vi "Wormgear.vi"(8 "error in (no error)":errorcluster, 11 "Buttons":bool[](array[boolean])) -> (0 "error out":errorcluster, 3 "Wormgear Power":dbl)   [LabVIEW 2016]
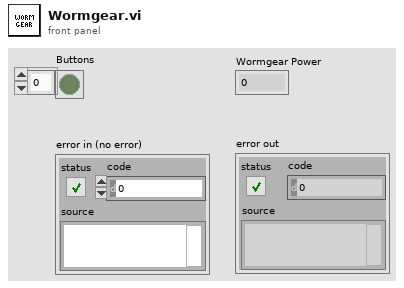
[diagram p1: front panel]
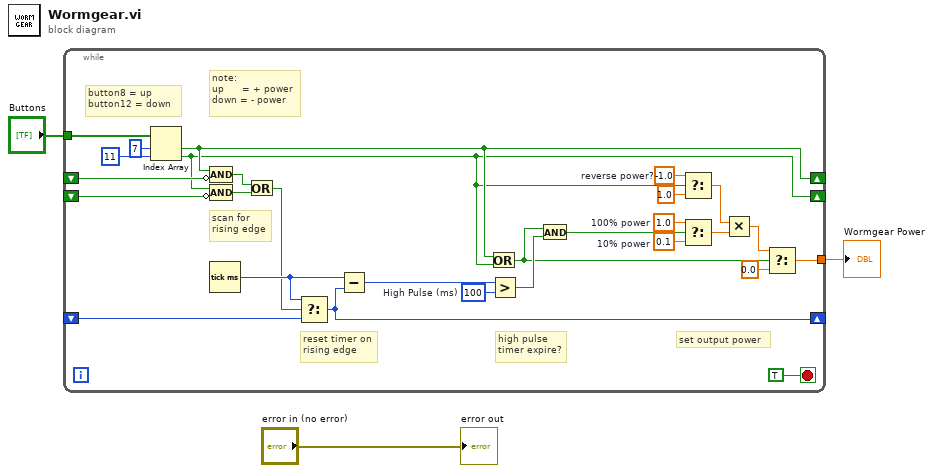
[diagram p0: block diagram]
diagram:
  n1 = while {
    tunnel: "Buttons" -> [w31]
    shift-right: [w5] -> _
    shift-left: _ -> [w28]
    shift-right: [w4] -> _
    shift-left: _ -> [w27]
    shift-right: [w22] -> _
    shift-left: _ -> [w24]
    tunnel: [w7] -> w2
    stop <- TRUE stop-if-true
    w14 = -1.0  # reverse power?
    w15 = 0.1  # 10% power
    w16 = 1.0  # 100% power
    w20 = u32 100  # High Pulse (ms)
    # "set output power"
    # "high pulse\ntimer expire?"
    # "note:\nup      = + power\ndown = - power"
    # "reset timer on\nrising edge"
    # "scan for\nrising edge"
    # "button8 = up\nbutton12 = down"
    n2 = Index Array(array=w31, index #1=7 ("index"), index #2=11 ("index")) -> (element #1=w5:bool, element #2=w4:bool)
    n3 = Compound Arithmetic op=AND(w5, invert w28) -> (w26:bool)
    n4 = Compound Arithmetic op=AND(w4, invert w27) -> (w25:bool)
    n5 = Tick Count (ms)() -> (millisecond timer value=w23:u32)
    n6 = Or(x=w26, y=w25) -> (x .or. y?=w19:bool)
    n7 = Select(t=w23, s=w19, f=w24) -> (s? t:f=w22:u32)
    n8 = Subtract(x=w23, y=w22) -> (x-y=w21:u32)
    n9 = Or(x=w5, y=w4) -> (x .or. y?=w10:bool)
    n10 = Greater?(x=w21, y=w20) -> (0:w18:bool)
    n11 = And(x=w10, y=w18) -> (x .and. y?=w17:bool)
    n12 = Select(t=w14, s=w4, f=1.0) -> (s? t:f=w11:dbl)
    n13 = Select(t=w16, s=w17, f=w15) -> (s? t:f=w12:dbl)
    n14 = Multiply(x=w11, y=w12) -> (x*y=w9:dbl)
    n15 = Select(t=w9, s=w10, f=0.0) -> (s? t:f=w7:dbl)
  }
  "Wormgear Power" <- w2
  "error out" <- "error in (no error)"
